vi "tracking and stage files global.vi"() -> ()   [LabVIEW 2010]
panel:
  out "auto-record":bool=TRUE
  out "record":bool
  in  "record stage":bool=TRUE
  in  "record tracking":bool=TRUE
  in  "stub":string="lineName"
  in  "base directory":path
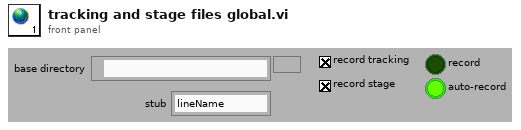
[diagram p1: front panel]
diagram:
